vi "_CSMObj-Information.vi"(7 "Allowed Messages (Empty For All)":string[](array[string]), 8 "Error In":errorcluster caption="error in (no error)", 11 "Requested Name":string) -> (0 "error out":errorcluster, 3 "CSMO-Info":T1)   [LabVIEW 2017, in "Communicable State Machine.lvlib"]
uses:
  Communicable State Machine.lvlib
  _CSMObj-Info.ctl
  Typedef/_CSM_MODE.ctl
  _Shared/CSM Shared.lvlib
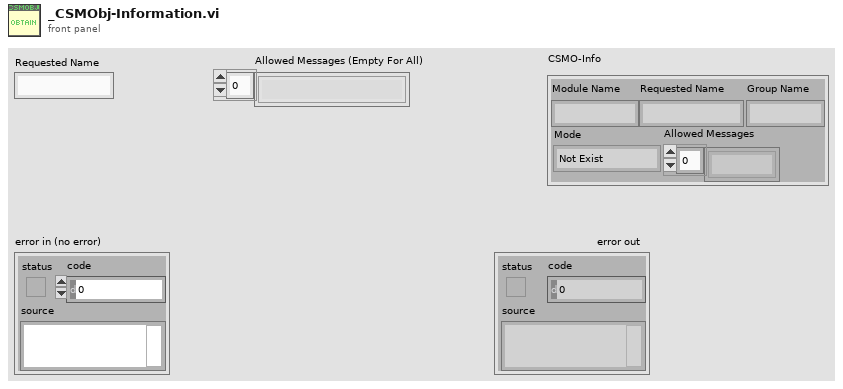
[diagram p1: front panel]
types:
  T1 = typedef "Communicable State Machine.lvlib/_CSMObj-Info.ctl" = cluster{"Module Name":string, "Requested Name":string, "Group Name":string, "Mode":T2, "Allowed Messages":string[]}
  T2 = typedef "Communicable State Machine.lvlib/_CSM_MODE.ctl" = enum16{"Not Exist", "Stand Alone", "CSM", "Worker", "Worker Agent", "Chain Node", "Chain"}
  T3 = typedef "Communicable State Machine.lvlib/_CSM_NAME_REQUEST.ctl" = enum16{"Stand Alone CSM Request", "Normal CSM Request", "Agent Request", "Action Worker Request", "Chain Request", "Chain Node Request"}
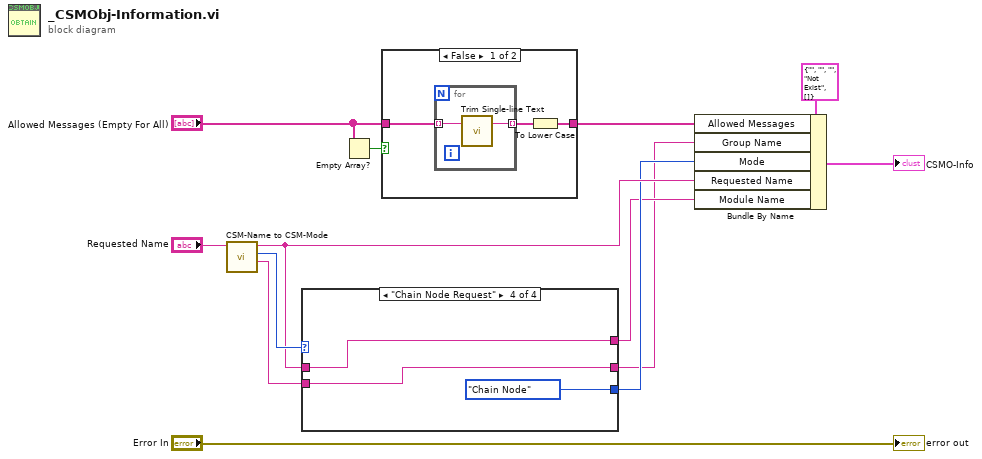
[diagram p0: block diagram]
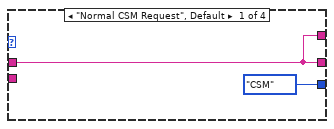
[diagram p2: hidden frame]
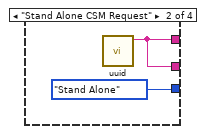
[diagram p3: hidden frame]
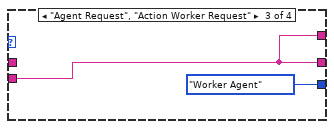
[diagram p4: hidden frame]
diagram:
  n1 = call "CSM-Name to CSM-Mode.vi"("String"="Requested Name") -> ("ParentCSM Name"=w8:string, "CSM Mode"=w6:T3, "Requested Name"=w5:string)  [unwired: 8 in]
  n2 = case shown="\"Chain Node Request\"" w6 {
    tunnel: [w14 w16 w18 w20] -> w2
    tunnel: w5 -> [w14 _ _ w21]
    tunnel: w8 -> [_ _ w18 w20]
    tunnel: [_CSM_MODE."CSM" ("Mode") _CSM_MODE."Stand Alone" ("Mode") _CSM_MODE."Worker Agent" ("Mode") _CSM_MODE."Chain Node" ("Mode")] -> w4
    tunnel: [w14 w16 w18 w21] -> w3
    frame "Normal CSM Request", Default {
    }
    frame "Stand Alone CSM Request" {
      n3 = call "uuid.vi"() -> ("UUID"=w16:string)  [unwired: 11 in]
    }
    frame "Agent Request", "Action Worker Request" {
    }
    frame "Chain Node Request" {
    }
  }
  n4 = Empty Array?(array="Allowed Messages (Empty For All)") -> (empty?=w9:bool)
  n5 = case shown="False" w9 {
    tunnel: [w23 w28] -> w11
    tunnel: "Allowed Messages (Empty For All)" -> [w24 w28]
    frame False {
      n6 = for {
        tunnel: [w26] -> w25 mode=indexing
        tunnel: w24 -> [w27] mode=indexing
        n7 = call "Trim Single-line Text.vi"("single-line text"=w27) -> ("trimed text"=w26:string)  [unwired: 2 in]
      }
      n8 = To Lower Case(string=w25) -> (all lower case string=w23:string[])
    }
    frame True {
    }
  }
  n9 = Bundle By Name(cluster=T1 {"Module Name"="", "Requested Name"="", "Group Name"="", "Mode"=enum."Not Exist", "Allowed Messages"=[]} ("CSMQ in"), "Allowed Messages"=w11, "Group Name"=w2, "Mode"=w4, "Requested Name"=w5, "Module Name"=w3) -> (→"CSMO-Info":T1)
  "error out" <- "Error In"
